vi "SR430.set trig offset.vi"(0 "i ref in":refnum<vi>, 2 "triggerOffset":i32, 3 "ms timeout (10000)":i32=10000, 5 "error in (no error)":errorcluster) -> (14 "i ref out":refnum<vi>, 17 "timed out":bool, 19 "error out":errorcluster)   [LabVIEW 2014, in "SR430.lvlib"]
doc: "Sets the Trigger Offset.\nThe value can go from 0 to 16384 per step of 16."
uses:
  SR430.lvlib
  CS_Core/CSSystem/CoreDefs/CoreDefs.error_type.ctl
  instr.lib/SR430/SR430Driver.lvlib
  CS_Core/CSSystem/CoreLib/CoreLib.lvlib
  CSlibraries/UtilityLib/UtilityLib.lvlib
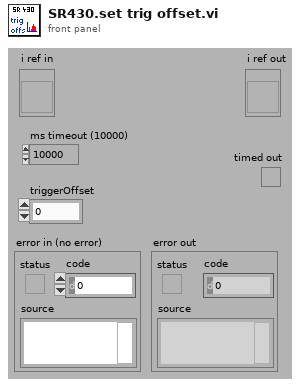
[diagram p1: front panel]
types:
  T1 = typedef "CoreDefs.error_type.ctl" = enum16{"no error", "can't load process", "can't unload process", "process does not exist", "can't install process", "can't remove process", "unknown function", "time out", "can't execute function", "duplicate queue name", "super not found", "caller queue invalid", "can't ping process", "unknown error", "VISA Error", "VISA timeout", "GPIB timeout", "GPIB error", "communication error", "data type mismatch", "can't read data from OPC server", "can't write data to OPC server", "OET error", "function not implemented", "process already exists", "invalid Shared Variable name", "error writing Shared Variable", "error reading Shared Variable", "invalid client name", "corrupt database", "unknown class", "call not authorized", "parameter out of range", "OET timeout: can't get data to modify", "invalid queue name", "requested operation incompatible with current state", "event undefined", "event disabled", "state undefined", "caller is not a friend", "EventBuilder: bad eventID", "EventBuilder: no DAQ devices", "a thread must not stop itself", "UNUSED ELEMENT4", "DiscArchiver: eventData incomplete", "DiscArchiver: eventData does not belong to run", "DiscArchiver: can't open file", "DiscArchiver: can't write to file", "DiscArchiver: available disc space low", "can't acquire semaphore", "error reading data from database", "notifier object is not existing", "can't register process", "can't unregister process", "illegal event type", "object disabled", "object already exists", "can't change state", "Instrument not found", "no connection to remote node", "invalid reference", "N/A", "UNUSED ELEMENT 1", "element not found", "illegal TCP/IP connection detected", "object does not exist", "invalid access ID", "unknown CS system", "invalid privilige", "unsupported data type", "unsupported server type", "IO server already exists", "Shared Variable already exists"}
  T2 = typedef "SR430Driver.lvlib/SR430_VISA Control.ctl" = cluster{"VISA resource name":refnum<visa-resource-name>}
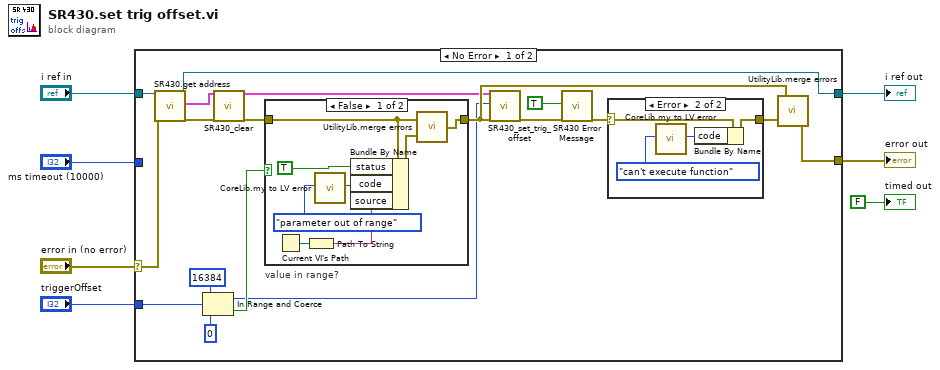
[diagram p0: block diagram]
diagram:
  n1 = case shown="No Error" "error in (no error)" {
    selector: "error in (no error)" -> [w8 w40]
    tunnel: "i ref in" -> [w25 w41]
    tunnel: "triggerOffset" -> [w22 _]
    tunnel: [w21 w40] -> w5
    tunnel: [w20 w41] -> w4
    tunnel: "ms timeout (10000)" -> [_ _]
    frame No Error {
      n2 = call "SR430.get address.vi"("i ref in"=w25, "error in (no error)"=w8) -> ("i ref out"=w20:refnum<vi>, "address"=w24:T2, "error out"=w23:errorcluster)  [unwired: 15 in]
      n3 = In Range and Coerce(upper limit=16384, x=w22, lower limit=0) -> (coerced(x)=w14:i32, In Range?=w15:bool)
      n4 = call "SR430_clear.vi"("address"=w24, "error in (no error)"=w23) -> ("address out"=w10:T2, "error out"=w9:errorcluster)  [unwired: 16 in]
      n5 = case "value in range?" shown="False" w15 {
        tunnel: w9 -> [w27 w34]
        tunnel: [w30 w34] -> w17
        frame False {
          n6 = Current VI's Path() -> (path=w29:path)
          n7 = Path To String(path=w29) -> (string=w28:string)
          n8 = call "CoreLib.my to LV error.vi"("ErrorTypes"=CoreDefs.error_type."parameter out of range") -> ("LV error code"=w32:i32)  [unwired: 17 in, 1 out]
          n9 = Bundle By Name(cluster=w27, "status"=TRUE, "code"=w32, "source"=w28) -> (w26:errorcluster)
          n10 = call "UtilityLib.merge errors.vi"("error2 (no error)"=w26, "error1 (no error)"=w27) -> ("error out"=w30:errorcluster)
        }
        frame True {
        }
      }
      n11 = call "SR430_set_trig_offset.vi"("address"=w10, "triggerOffset"=w14, "error in (no error)"=w17) -> ("error out"=w11:errorcluster)  [unwired: 15 in, 1 out]
      n12 = call "SR430 Error Message.vi"("addMessageToSource"=TRUE ("add message to source"), "error in (no error)"=w11) -> ("error out"=w19:errorcluster)  [unwired: 14 in, 3 out]
      n13 = case shown="Error" w19 {
        selector: w19 -> [w35 w39]
        tunnel: [w35 w36] -> w16
        frame No Error {
        }
        frame Error {
          n14 = call "CoreLib.my to LV error.vi"("ErrorTypes"=CoreDefs.error_type."can't execute function") -> ("LV error code"=w38:i32)  [unwired: 17 in, 1 out]
          n15 = Bundle By Name(cluster=w39, "code"=w38) -> (w36:errorcluster)
        }
      }
      n16 = call "UtilityLib.merge errors.vi"("error2 (no error)"=w16, "error1 (no error)"=w17) -> ("error out"=w21:errorcluster)
    }
    frame Error {
    }
  }
  "error out" <- w5
  "i ref out" <- w4
  "timed out" <- FALSE ("timed out")
